vi "shouldWater.vi"(5 "SoilVeryDry":dbl=20.0, 6 "Night Light":dbl=15.0, 7 "SoilDry":dbl=30.0, 8 "lightLevel":dbl, 9 "soilMoist":dbl, 10 "airRH":dbl, 11 "tempC":dbl) -> (2 "shouldWater":bool)   [LabVIEW 2025]
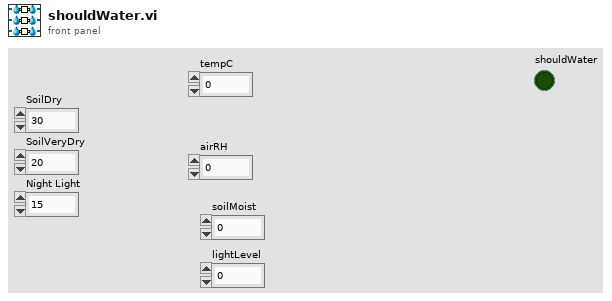
[diagram p1: front panel]
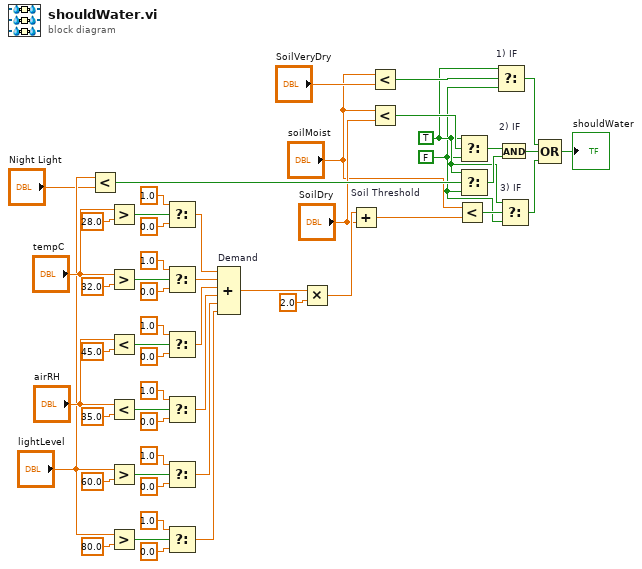
[diagram p0: block diagram]
diagram:
  w1 = FALSE
  w6 = TRUE
  n1 = Less?(x="lightLevel", y="Night Light") -> (x < y?=w14:bool)
  n2 = Greater?(x="tempC", y=28.0) -> (0:w43:bool)
  n3 = Greater?(x="tempC", y=32.0) -> (0:w38:bool)
  n4 = Less?(x="airRH", y=45.0) -> (x < y?=w35:bool)
  n5 = Less?(x="airRH", y=35.0) -> (x < y?=w32:bool)
  n6 = Greater?(x="lightLevel", y=60.0) -> (0:w29:bool)
  n7 = Greater?(x="lightLevel", y=80.0) -> (0:w26:bool)
  n8 = Select(t=1.0, s=w43, f=0.0) -> (s? t:f=w25:dbl)
  n9 = Select(t=1.0, s=w38, f=0.0) -> (s? t:f=w24:dbl)
  n10 = Select(t=1.0, s=w35, f=0.0) -> (s? t:f=w23:dbl)
  n11 = Select(t=1.0, s=w32, f=0.0) -> (s? t:f=w22:dbl)
  n12 = Select(t=1.0, s=w29, f=0.0) -> (s? t:f=w21:dbl)
  n13 = Select(t=1.0, s=w26, f=0.0) -> (s? t:f=w20:dbl)
  n14 = Compound Arithmetic op=ADD "Demand"(w25, w24, w23, w22, w21, w20) -> (w19:dbl)
  n15 = Multiply(x=w19, y=2.0) -> (x*y=w44:dbl)
  n16 = Add "Soil Threshold"(x=w44, y="SoilDry") -> (x+y=w8:dbl)
  n17 = Less?(x="soilMoist", y="SoilVeryDry") -> (x < y?=w17:bool)
  n18 = Less?(x="soilMoist", y="SoilDry") -> (x < y?=w12:bool)
  n19 = Less?(x="soilMoist", y=w8) -> (x < y?=w7:bool)
  n20 = Select(t=w6, s=w12, f=w1) -> (s? t:f=w11:bool)
  n21 = Select(t=w6, s=w14, f=w1) -> (s? t:f=w10:bool)
  n22 = Select "1) IF"(t=w6, s=w17, f=w1) -> (s? t:f=w5:bool)
  n23 = And "2) IF"(x=w11, y=w10) -> (x .and. y?=w4:bool)
  n24 = Select "3) IF"(t=w6, s=w7, f=w1) -> (s? t:f=w3:bool)
  n25 = Compound Arithmetic op=OR(w5, w4, w3) -> (→"shouldWater":bool)
